vi "Check File Properties.vi"(9 "Create if Non Existent?":bool, 10 "Read-Only?":bool, 11 "filepath":path) -> (0 "error out":errorcluster, 1 "File exists":bool, 2 "Read-Only":bool, 3 "filepath dup":path, 4 "is Directory":bool)   [LabVIEW 2013, in "CfgManager.Text.lvlib" / "ConfigManager.Text.lvclass"]
uses:
  ConfigManager.Text.lvclass
  <vilib>/Utility/error.llb/Error Cluster From Error Code.vi
  <vilib>/ErrorRing/Error Ring.xnode
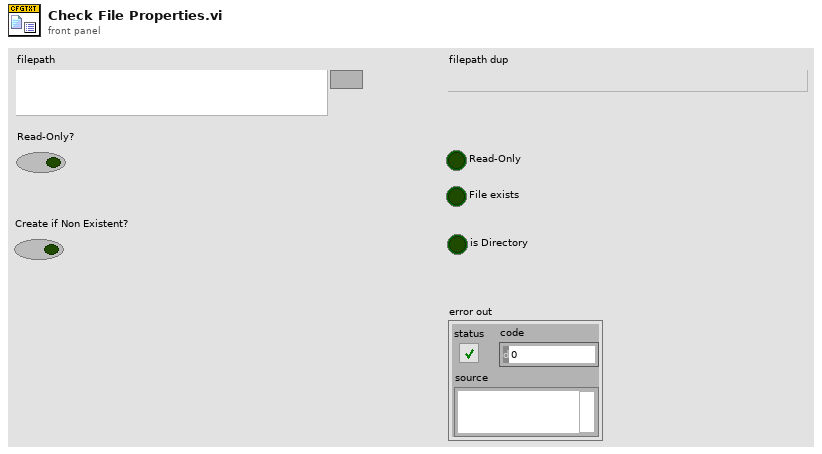
[diagram p1: front panel]
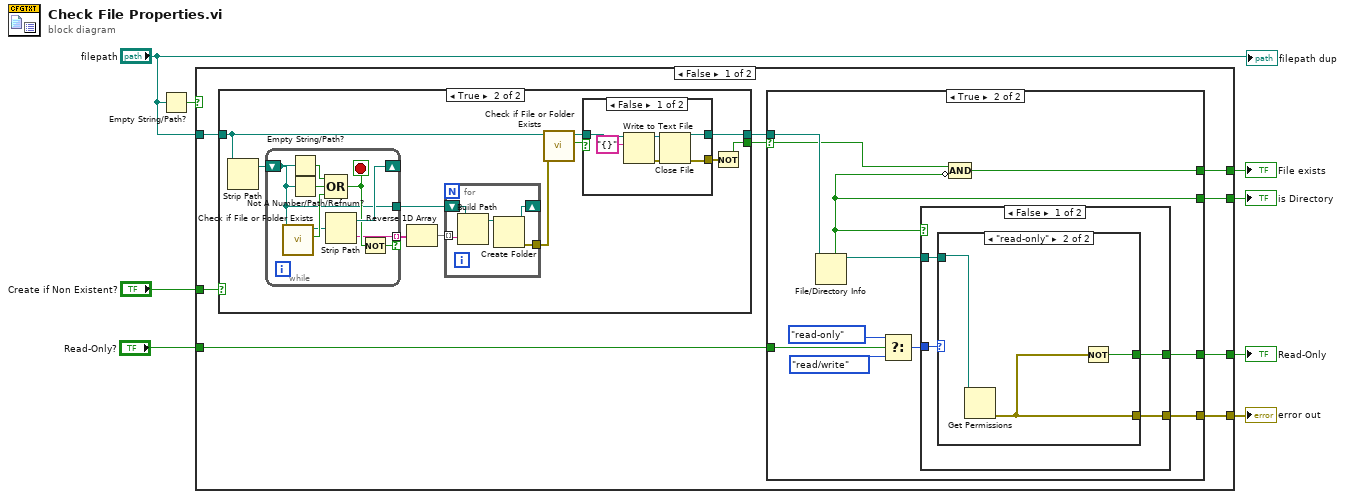
[diagram p0: block diagram]
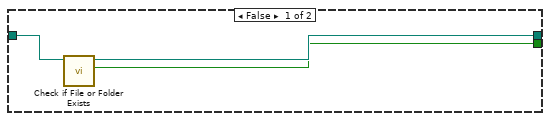
[diagram p2: hidden frame]
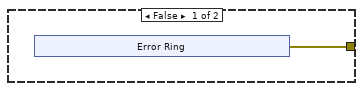
[diagram p4: hidden frame]
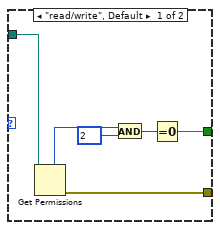
[diagram p5: hidden frame]
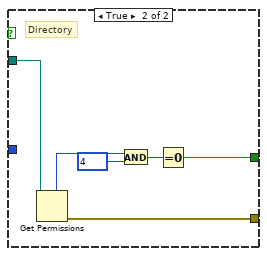
[diagram p6: hidden frame]
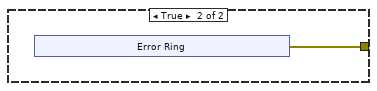
[diagram p7: hidden frame]
diagram:
  n1 = Empty String/Path?(string/path="filepath") -> (empty?=w3:bool)
  n2 = case shown="False" w3 {
    tunnel: [w17 _] -> w8
    tunnel: "Read-Only?" -> [w9 _]
    tunnel: [w16 _] -> w6
    tunnel: [w15 _] -> w5
    tunnel: "filepath" -> [w13 _]
    tunnel: [w14 w88] -> w2
    tunnel: "Create if Non Existent?" -> [w10 _]
    frame False {
      n3 = case shown="True" w10 {
        tunnel: w13 -> [w20 w22]
        tunnel: [w19 w26] -> w12
        tunnel: [w18 w24] -> w11
        frame False {
          n4 = call <vilib>:"Check if File or Folder Exists.vi"("path"=w20) -> ("file or folder exists?"=w18:bool, "dup path"=w19:path)  [unwired: 8 in, 1 out]
        }
        frame True {
          n5 = Strip Path(path=w22) -> (stripped path=w29:path)  [unwired: 1 out]
          n6 = while {
            shift-right: [w52] -> _
            shift-left: w29 -> [w44]
            tunnel: [w47] -> w31 mode=indexing if=w48
            tunnel: [w44] -> w23
            stop <- w49 stop-if-true
            n7 = call <vilib>:"Check if File or Folder Exists.vi"("path"=w44) -> ("file or folder exists?"=w46:bool, "dup path"=w45:path)  [unwired: 8 in, 1 out]
            n8 = Empty String/Path?(string/path=w44) -> (empty?=w50:bool)
            n9 = Not A Number/Path/Refnum?(number/path/refnum=w44) -> (NaN/Path/Refnum?=w51:bool)
            n10 = Compound Arithmetic op=OR(w50, w51, w46) -> (w49:bool)
            n11 = Strip Path(path=w45) -> (stripped path=w52:path, name=w47:string)
            n12 = Not(x=w49) -> (.not. x?=w48:bool)
          }
          n13 = Reverse 1D Array(array=w31) -> (reversed array=w30:string[])
          n14 = for {
            tunnel: w30 -> [w42] mode=indexing
            shift-right: [w39] -> _
            shift-left: w23 -> [w43]
            tunnel: [w40] -> w21
            n15 = Build Path(base path=w43, name or relative path=w42) -> (appended path=w41:path)
            n16 = Create Folder(path (use dialog)=w41) -> (created path=w39:path, error out=w40:errorcluster)  [unwired: 2 in, 1 out]
          }
          n17 = call <vilib>:"Check if File or Folder Exists.vi"("error in (no error)"=w21, "path"=w22) -> ("file or folder exists?"=w28:bool, "dup path"=w27:path)  [unwired: 7 in, 1 out]
          n18 = case shown="False" w28 {
            tunnel: w27 -> [w37 w38]
            tunnel: [w33 w38] -> w26
            tunnel: [w32 _] -> w25
            frame False {
              n19 = Write to Text File(file (use dialog)=w37, text="{}") -> (refnum out=w34:refnum<file>, error out=w35:errorcluster)  [unwired: 2 in, 1 out]
              n20 = Close File(refnum=w34, error in=w35) -> (path=w33:path, error out=w32:errorcluster)
            }
            frame True {
            }
          }
          n21 = Not(x=w25) -> (.not. x?=w24:bool)
        }
      }
      n22 = case shown="True" w11 {
        selector: w11 -> [_ w58]
        tunnel: [_ w68] -> w17
        tunnel: w9 -> [_ w67]
        tunnel: [_ w63] -> w16
        tunnel: [_ w62] -> w15
        tunnel: [w53 w60] -> w14
        tunnel: w12 -> [_ w59]
        frame False {
          n23 = xnode "Error Ring"() -> ("error out"=w53:errorcluster)
        }
        frame True {
          n24 = File/Directory Info(path=w59) -> (path out=w61:path, directory=w62:bool)  [unwired: 1 in, 5 out]
          n25 = Select(t=enum16{"read/write", "read-only", "write-only"}."read-only" ("access (0:read/write)"), s=w67, f=enum16{"read/write", "read-only", "write-only"}."read/write" ("access (0:read/write)")) -> (s? t:f=w64:enum16{"read/write", "read-only", "write-only"})
          n26 = case shown="False" w62 {
            tunnel: w64 -> [w72 _]
            tunnel: [w71 w83] -> w63
            tunnel: w61 -> [w70 w87]
            tunnel: [w69 w82] -> w60
            frame False {
              n27 = case shown="\"read-only\"" w72 {
                tunnel: [w73 w80] -> w71
                tunnel: w70 -> [w75 w81]
                tunnel: [w74 w79] -> w69
                frame "read/write", Default {
                  n28 = Get Permissions(11:w75) -> (0:w74:errorcluster, 5:w78:i16)  [unwired: 1 in, 3 out]
                  n29 = And(x=w78, y=i16 2) -> (x .and. y?=w76:i16)
                  n30 = Equal To 0?(x=w76) -> (x = 0?=w73:bool)
                }
                frame "read-only" {
                  n31 = Get Permissions(11:w81) -> (0:w79:errorcluster)  [unwired: 1 in, 4 out]
                  n32 = Not(x=w79) -> (.not. x?=w80:bool)
                }
              }
            }
            frame True {
              # "Directory"
              n33 = Get Permissions(11:w87) -> (0:w82:errorcluster, 5:w86:i16)  [unwired: 1 in, 3 out]
              n34 = And(x=w86, y=i16 4) -> (x .and. y?=w84:i16)
              n35 = Equal To 0?(x=w84) -> (x = 0?=w83:bool)
            }
          }
          n36 = Compound Arithmetic op=AND(w58, invert w62) -> (w68:bool)
        }
      }
    }
    frame True {
      n37 = xnode "Error Ring"() -> ("error out"=w88:errorcluster)
    }
  }
  "Read-Only" <- w6
  "File exists" <- w8
  "is Directory" <- w5
  "error out" <- w2
  "filepath dup" <- "filepath"
